vi "SLMControl_LabView.vi"() -> ()   [LabVIEW 2022 SP3]
panel:
  in  "SLM Driver":bool
  out "SLM Driver Error":errorcluster
  in  "Loop":bool
  in  "Array":dbl[][](array[numeric])
  out "Array output":dbl[][](array[numeric]) format="%#_13g"
  out "Pattern Generator Error":errorcluster
  in  "Python file path":path
  out "Intensity Graph":dbl[][](graph)
  in  "deflect_angle":dbl
  in  "lens_size":u16
  in  "offset_x":i8(slide) scale=0.0..20.0
  in  "offset_y":i8(slide) scale=0.0..20.0
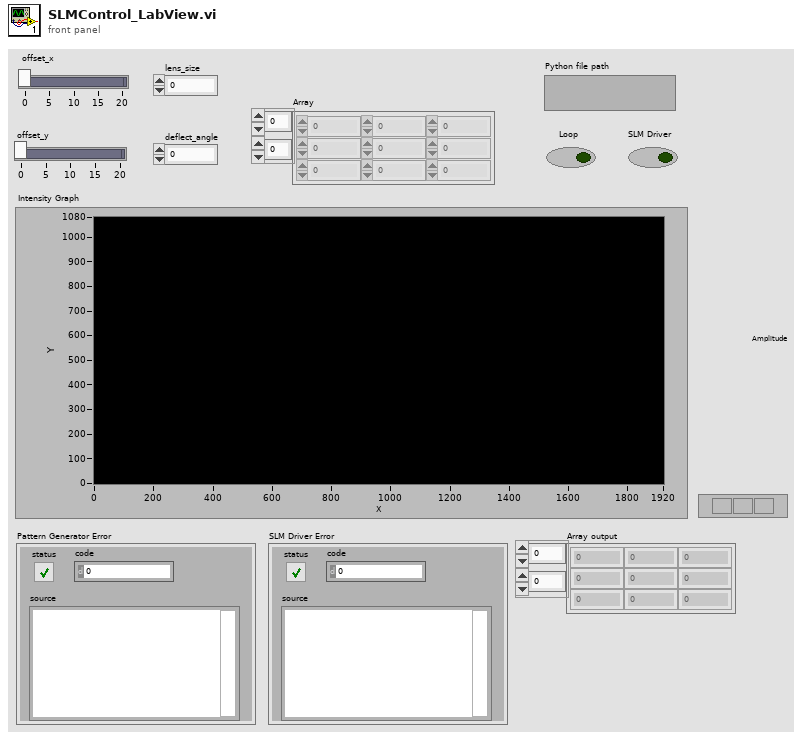
[diagram p1: front panel]
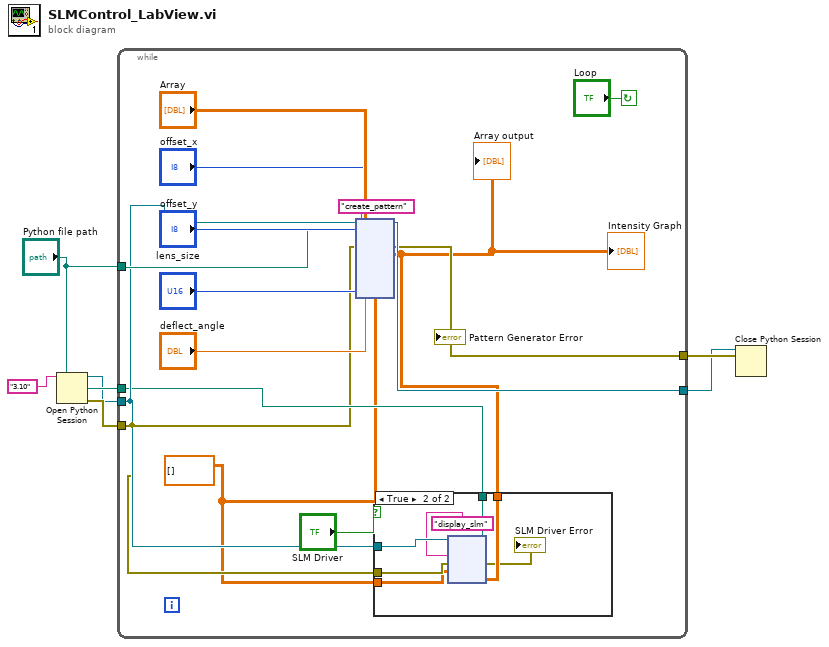
[diagram p0: block diagram]
diagram:
  n1 = Open Python Session(python version="3.10") -> (session out=w1:refnum<k35>, error out=w6:errorcluster)  [unwired: 2 in]
  n2 = while {
    tunnel: w6 -> [w10]
    tunnel: [w13] -> w4
    tunnel: [w16] -> w3
    tunnel: "Python file path" -> [w15]
    tunnel: "Python file path" -> [w11]
    tunnel: w1 -> [w12]
    stop <- "Loop" continue-if-true
    w9 = dbl[][] []
    n3 = node(w12, w15, "create_pattern", w10, w9, "Array", "offset_x", "offset_y", "lens_size", "deflect_angle") -> (w16:refnum<k35>, w13:errorcluster, w7:dbl[][])  [unwired: 5 in, 2 out]
    "Intensity Graph" <- w7
    "Array output" <- w7
    "Pattern Generator Error" <- w13
    n4 = case shown="True" "SLM Driver" {
      tunnel: w12 -> [_ w29]
      tunnel: w11 -> [_ w28]
      tunnel: w10 -> [_ w27]
      tunnel: w9 -> [_ w26]
      tunnel: w7 -> [_ w25]
      frame False {
      }
      frame True {
        n5 = node(w29, w28, "display_slm", w27, w26, w25) -> (→"SLM Driver Error":errorcluster)  [unwired: 2 in, 3 out]
      }
    }
  }
  n6 = Close Python Session(session in=w3, error in=w4) -> ()  [unwired: 1 out]
